vi "Change_Circuit_Mode.vi"(8 "Error In":errorcluster, 9 "Circuit Mode\n1, Auto\n2, Series\n3, Parallel":i32) -> (0 "error out":errorcluster)   [LabVIEW 2020]
panel:
  in  "Input String":string
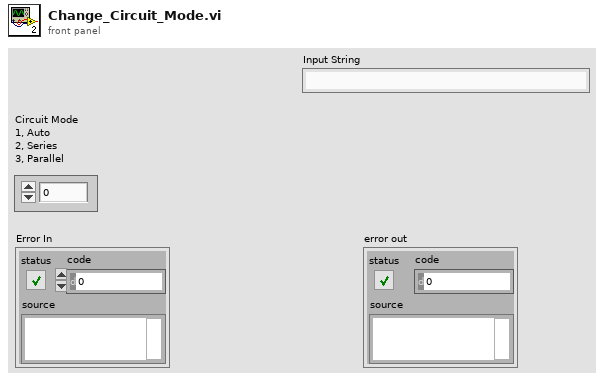
[diagram p1: front panel]
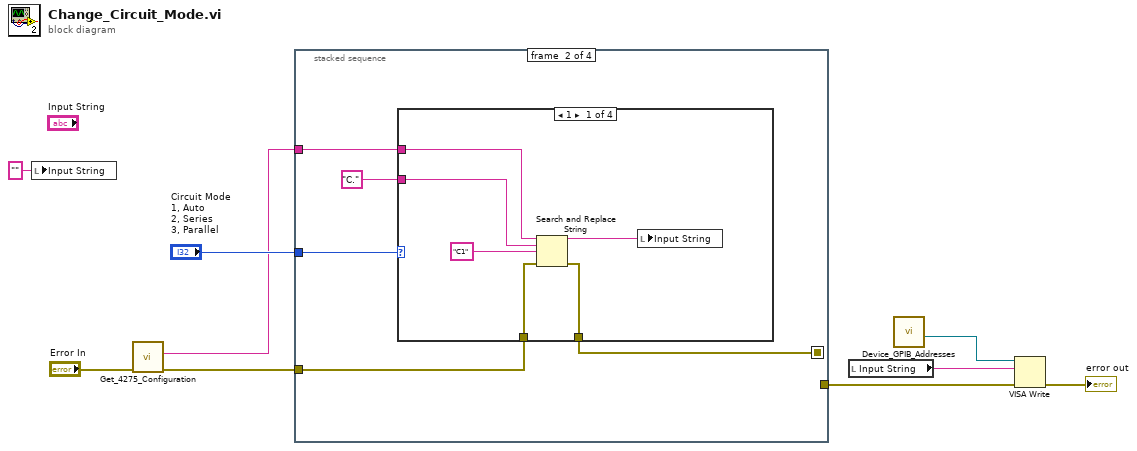
[diagram p0: block diagram]
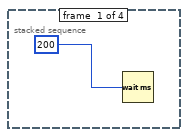
[diagram p2: hidden frame]
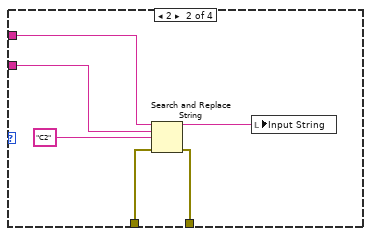
[diagram p3: hidden frame]
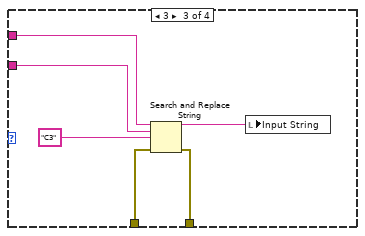
[diagram p4: hidden frame]
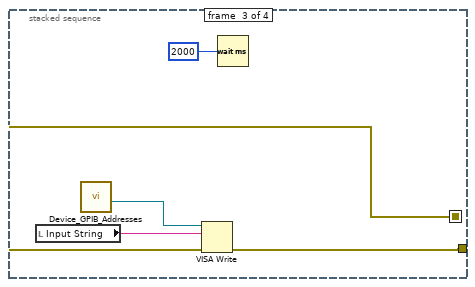
[diagram p6: hidden frame]
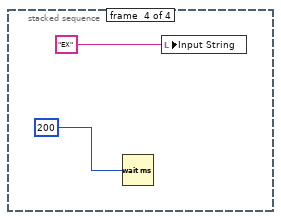
[diagram p7: hidden frame]
diagram:
  n1 = local write "Input String"("" ("Input String")) -> ()
  n2 = call "Get_4275_Configuration.vi"("error in"="Error In") -> ("error out"=w7:errorcluster, "Keystate"=w6:string)  [unwired: 9 in]
  n3 = stacked-sequence {
    seq-local: [_ w11 _ _] -> [_ _ w36 _]
    tunnel: "Circuit Mode\n1, Auto\n2, Series\n3, Parallel" -> [_ w15 _ _]
    tunnel: w7 -> [_ w14 _ _]
    tunnel: w6 -> [_ w13 _ _]
    tunnel: [_ _ w35 _] -> w3
    frame #0 {
      n4 = Wait (ms)(milliseconds to wait=u32 200) -> ()  [unwired: 1 out]
    }
    frame #1 {
      n5 = case shown="1" w15 {
        tunnel: w14 -> [w21 w25 w32 w34]
        tunnel: w13 -> [w20 w26 w31 _]
        tunnel: [w18 w24 w30 w34] -> w11
        tunnel: "C." ("search string") -> [w17 w23 w29 _]
        frame 1 {
          n6 = Search and Replace String(input string=w20, search string=w17, replace string="C1" ("replace string (\"\")"), error in=w21) -> (result string=w16:string, error out=w18:errorcluster)  [unwired: 4 in, 2 out]
          n7 = local write "Input String"(w16) -> ()
        }
        frame 2 {
          n8 = Search and Replace String(input string=w26, search string=w23, replace string="C2" ("replace string (\"\")"), error in=w25) -> (result string=w22:string, error out=w24:errorcluster)  [unwired: 4 in, 2 out]
          n9 = local write "Input String"(w22) -> ()
        }
        frame 3 {
          n10 = Search and Replace String(input string=w31, search string=w29, replace string="C3" ("replace string (\"\")"), error in=w32) -> (result string=w28:string, error out=w30:errorcluster)  [unwired: 4 in, 2 out]
          n11 = local write "Input String"(w28) -> ()
        }
        frame Default {
        }
      }
    }
    frame #2 {
      n12 = local read "Input String"() -> (w38:string)
      n13 = call "Device_GPIB_Addresses.vi"() -> ("HP 4275A Address"=w37:refnum<visa-resource-name>)  [unwired: 9 in, 2 out]
      n14 = VISA Write(VISA resource name=w37, write buffer=w38, error in (no error)=w36) -> (error out=w35:errorcluster)  [unwired: 2 out]
      n15 = Wait (ms)(milliseconds to wait=u32 2000) -> ()  [unwired: 1 out]
    }
    frame #3 {
      n16 = Wait (ms)(milliseconds to wait=u32 200) -> ()  [unwired: 1 out]
      n17 = local write "Input String"("EX" ("Input String")) -> ()
    }
  }
  n18 = local read "Input String"() -> (w4:string)
  n19 = call "Device_GPIB_Addresses.vi"() -> ("HP 4275A Address"=w5:refnum<visa-resource-name>)  [unwired: 9 in, 2 out]
  n20 = VISA Write(VISA resource name=w5, write buffer=w4, error in (no error)=w3) -> (error out=→"error out":errorcluster)  [unwired: 2 out]
